vi "Page_Info_Read.vi"(6 "ctlReferences":T1, 8 "error in (no error)":errorcluster, 11 "AB_Build in":refnum<class "AB_Build.lvclass">) -> (0 "error out":errorcluster, 3 "AB_Build out":refnum<class "AB_Build.lvclass">)   [LabVIEW 2020, in "AB_Build.lvclass"]
uses:
  <vilib>/AppBuilder/AB_Classes/Build/AB_Build.lvclass
  <resource>/Framework/Providers/Builds/AppBuilder/AB_UI_Page_Info_References.ctl
  <vilib>/AppBuilder/AB_Classes/Build/AB_Build.lvclass/AB_Build.ctl
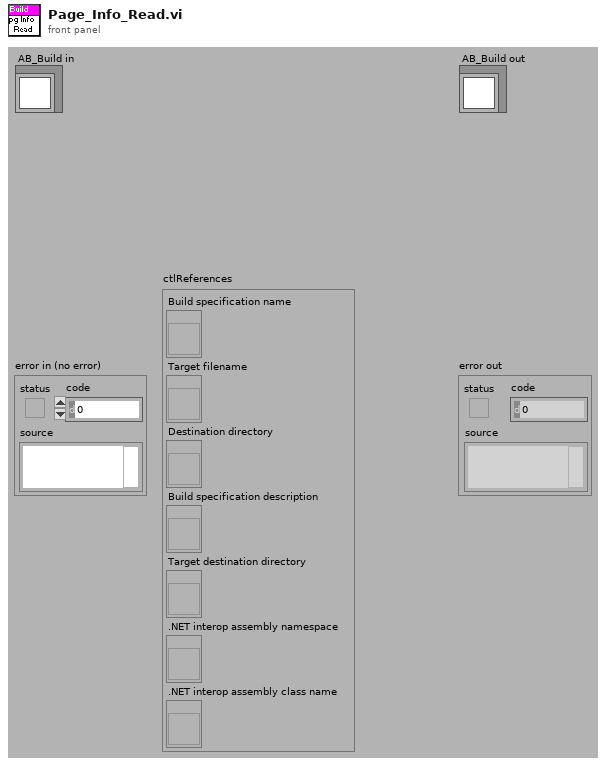
[diagram p1: front panel]
types:
  T1 = typedef "AB_UI_Page_Info_References.ctl" = cluster{"Build specification name":refnum<vi>, "Target filename":refnum<vi>, "Destination directory":refnum<vi>, "Build specification description":refnum<vi>, "Target destination directory":refnum<vi>, ".NET interop assembly namespace":refnum<vi>, ".NET interop assembly class name":refnum<vi>}
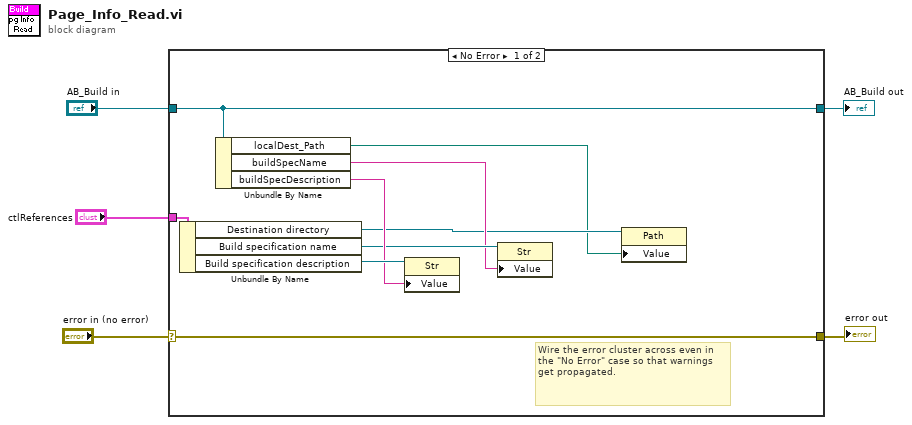
[diagram p0: block diagram]
diagram:
  n1 = case shown="No Error" "error in (no error)" {
    selector: "error in (no error)" -> [w14 w16]
    tunnel: [w14 w16] -> w4
    tunnel: [w13 w15] -> w2
    tunnel: "AB_Build in" -> [w13 w15]
    tunnel: "ctlReferences" -> [w12 _]
    frame No Error {
      # "Wire the error cluster across even in the \"No Error\" case so that warnings get propagated."
      n2 = Unbundle By Name(w12) -> ("Destination directory"=w7:refnum<vi>, "Build specification name"=w9:refnum<vi>, "Build specification description"=w11:refnum<vi>)
      n3 = Unbundle By Name(w13) -> ("localDest_Path"=w6:path, "buildSpecName"=w8:string, "buildSpecDescription"=w10:string)
      n4 = property class="Str"(reference=w11, "Value"=w10) -> ()  [unwired: 1 in, 2 out]
      n5 = property class="Str"(reference=w9, "Value"=w8) -> ()  [unwired: 1 in, 2 out]
      n6 = property class="Path"(reference=w7, "Value"=w6) -> ()  [unwired: 1 in, 2 out]
    }
    frame Error {
    }
  }
  "error out" <- w4
  "AB_Build out" <- w2
